vi "SRingStartThread.vi"(1 "releasems":i16=2, 2 "threadp":u32=31, 3 "ringdepth":u32) -> ()   [LabVIEW 2015]
uses:
  ESLSCDLL.dll
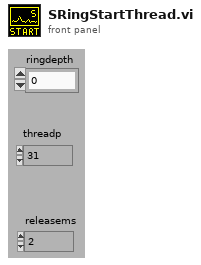
[diagram p1: front panel]
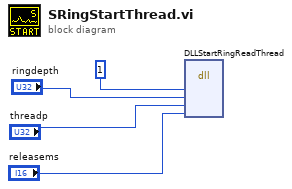
[diagram p0: block diagram]
diagram:
  n1 = dll-call lib="C:/ENTW/PCIE/64bit/lv64/1cam/board.vis/ESLSCDLL.dll" fn="DLLStartRingReadThread"("drv"=u32 1, "ringdepth"="ringdepth", "threadp"="threadp", "releasems"="releasems") -> ()  [unwired: 8 in, 2 out]
